vi "Insight_Send_Synch_Pulse_Wavelength.vi"(8 "error in (no error)":errorcluster, 9 "Mode (Read / Write)":enum8{"Write", "Read"}(ring), 10 "WL Pulse Parameters":T1={"FSR (GHz)"=1.0, "Delay (nsec)"=100.0, "Width (nsec)"=2.5}, 11 "telnet connection":T2) -> (0 "error out":errorcluster, 1 "response data":string, 2 "WL Pulse Parameters Out":T1, 3 "telnet  connection out":T2)   [LabVIEW 2015]
doc: "Insight Photonic Solutions\n\nThis VI generates a short wavelength pulse from the laser, for use in synchronizing the laser sweep with a data acquisition system that is measuring the signal from an interferometer. Based on the Free Spectral Range (FSR) of the interferometer, the wavelength step is FSR/4 to produce an amplitude change from the interferometer.\n\nInputs:\nRead/Write : query the pulse parameters or command the pulse to occur\nFSR (GHz) : the FSR of the interferometer, default 50 GHz.\nDelay (nsec) : 100 - 1000 nsec, default of 110 nsec.\n\nver 1.0 - original release\nver 1.9 - added width of pulse command\nver 3.3 - Parser now handles response from Atlas ver 3.2 and earlier, and Atlas 3.3 and later"
uses:
  Telnet Session.ctl
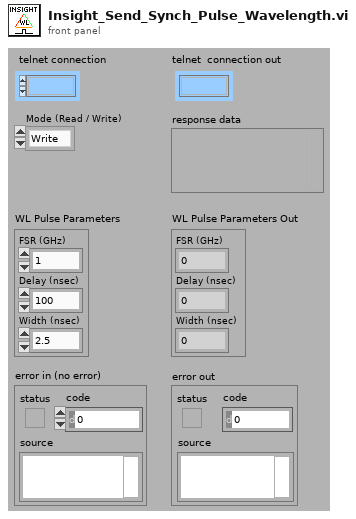
[diagram p1: front panel]
types:
  T1 = cluster{"FSR (GHz)":dbl, "Delay (nsec)":dbl, "Width (nsec)":dbl}
  T2 = typedef "Telnet Session.ctl" = refnum<k1>
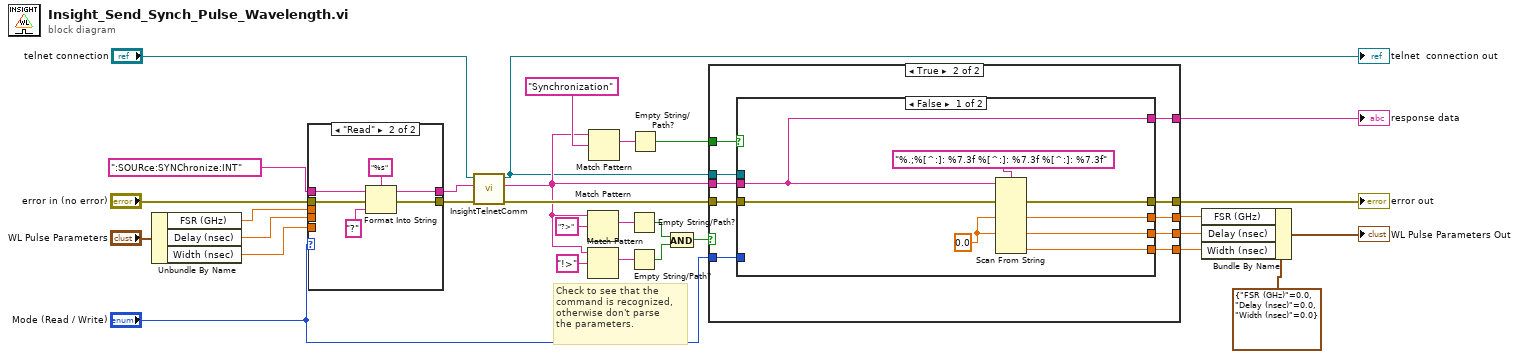
[diagram p0: block diagram]
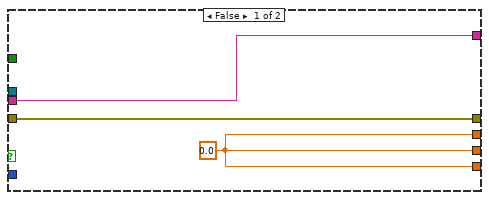
[diagram p2: hidden frame]
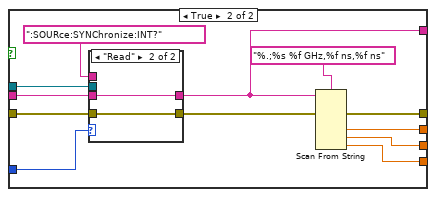
[diagram p3: hidden frame]
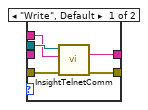
[diagram p4: hidden frame]
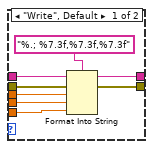
[diagram p5: hidden frame]
diagram:
  # "Check to see that the \ncommand is recognized,\notherwise don't parse \nthe parameters."
  n1 = Unbundle By Name("WL Pulse Parameters") -> ("FSR (GHz)"=w15:dbl, "Delay (nsec)"=w14:dbl, "Width (nsec)"=w9:dbl)
  n2 = case shown="\"Read\"" "Mode (Read / Write)" {
    tunnel: [w38 w40] -> w26
    tunnel: "error in (no error)" -> [w37 w39]
    tunnel: ":SOURce:SYNChronize:INT" ("String") -> [w36 w42]
    tunnel: w15 -> [w35 _]
    tunnel: [w33 w41] -> w29
    tunnel: w14 -> [w32 _]
    tunnel: w9 -> [w31 _]
    frame "Write", Default {
      n3 = Format Into String(format string="%.; %7.3f,%7.3f,%7.3f", initial string=w36, error in=w37, w35, w32, w31) -> (resulting string=w33:string, error out=w38:errorcluster)
    }
    frame "Read" {
      n4 = Format Into String(format string="%s", initial string=w42, error in=w39, "?" ("input 1")) -> (resulting string=w41:string, error out=w40:errorcluster)
    }
  }
  n5 = call "InsightTelnetComm.vi"("error in"=w26, "write buffer (\"\")"=w29, "telnet connection"="telnet connection") -> ("error out"=w24:errorcluster, "response data"=w5:string, "telnet  connection out"=w1:T2)  [unwired: 4 in]
  "telnet  connection out" <- w1
  n6 = Match Pattern(string=w5, regular expression="?>") -> (match substring=w22:string)  [unwired: 1 in, 3 out]
  n7 = Match Pattern(string=w5, regular expression="!>") -> (match substring=w21:string)  [unwired: 1 in, 3 out]
  n8 = Match Pattern(string=w5, regular expression="Synchronization") -> (match substring=w6:string)  [unwired: 1 in, 3 out]
  n9 = Empty String/Path?(string/path=w22) -> (empty?=w19:bool)
  n10 = Empty String/Path?(string/path=w21) -> (empty?=w18:bool)
  n11 = Empty String/Path?(string/path=w6) -> (empty?=w3:bool)
  n12 = And(x=w19, y=w18) -> (x .and. y?=w17:bool)
  n13 = case shown="True" w17 {
    tunnel: [w46 w57] -> w13
    tunnel: [w46 w56] -> w12
    tunnel: [w47 w55] -> w25
    tunnel: w24 -> [w47 w54]
    tunnel: w5 -> [w45 w53]
    tunnel: [w46 w52] -> w8
    tunnel: [w45 w50] -> w4
    tunnel: w3 -> [_ w51]
    tunnel: "Mode (Read / Write)" -> [_ w49]
    tunnel: w1 -> [_ w48]
    frame False {
      w46 = 0.0 ("default value 1")
    }
    frame True {
      n14 = case shown="False" w51 {
        tunnel: [w64 w68] -> w57
        tunnel: [w63 w67] -> w56
        tunnel: [w62 w76] -> w55
        tunnel: w54 -> [w61 w71]
        tunnel: w53 -> [w58 w73]
        tunnel: [w59 w66] -> w52
        tunnel: [w58 w69] -> w50
        tunnel: w49 -> [_ w74]
        tunnel: w48 -> [_ w70]
        frame False {
          w60 = 0.0 ("default value 1")
          n15 = Scan From String(format string="%.;%[^:]: %7.3f %[^:]: %7.3f %[^:]: %7.3f", input string=w58, error in=w61, default 2=w60, default 4=w60) -> (error out=w62:errorcluster, output 2=w64:dbl, output 4=w63:dbl, output 6=w59:dbl)  [unwired: 8 in, 2 out]
        }
        frame True {
          n16 = case shown="\"Read\"" w74 {
            tunnel: w71 -> [w82 w83]
            tunnel: [w81 w83] -> w72
            tunnel: w70 -> [w80 _]
            tunnel: ":SOURce:SYNChronize:INT?" ("String") -> [w79 _]
            tunnel: w73 -> [_ w84]
            tunnel: [w78 w84] -> w69
            frame "Write", Default {
              n17 = call "InsightTelnetComm.vi"("error in"=w82, "write buffer (\"\")"=w79, "telnet connection"=w80) -> ("error out"=w81:errorcluster, "response data"=w78:string)  [unwired: 4 in, 1 out]
            }
            frame "Read" {
            }
          }
          n18 = Scan From String(format string="%.;%s %f GHz,%f ns,%f ns", input string=w69, error in=w72) -> (error out=w76:errorcluster, output 2=w68:dbl, output 3=w67:dbl, output 4=w66:dbl)  [unwired: 6 in, 2 out]
        }
      }
    }
  }
  "error out" <- w25
  "response data" <- w4
  n19 = Bundle By Name(cluster=T1 {"FSR (GHz)"=0.0, "Delay (nsec)"=0.0, "Width (nsec)"=0.0} ("WL Pulse Parameters Out"), "FSR (GHz)"=w13, "Delay (nsec)"=w12, "Width (nsec)"=w8) -> (→"WL Pulse Parameters Out":T1)
